vi "CE14_open handshake(subVI).vi"(8 "error in(no error)":errorcluster, 11 "VISA resource name":refnum<visa-resource-name>) -> (0 "error out":errorcluster, 1 "success":bool, 2 "response msg":string[](array[string]), 3 "VISA resource name 2":refnum<visa-resource-name>)   [LabVIEW 2018, in "CE14_eMIC.lvlib"]
uses:
  CE14_eMIC.lvlib
  type defs/CE14_state.ctl
  <vilib>/Instr/_visa.llb/VISA Configure Serial Port (Instr).vi
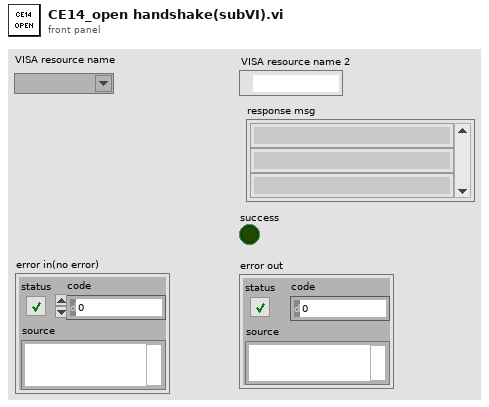
[diagram p1: front panel]
types:
  T1 = typedef "CE14_eMIC.lvlib/CE14_state.ctl" = enum16{"open COM (300)", "step1(300):2F 3F 21 0D 0A", "step2(300):06 30 34 31 0D 0A", "step3:Change4800", "step4(4800)", "stop"}
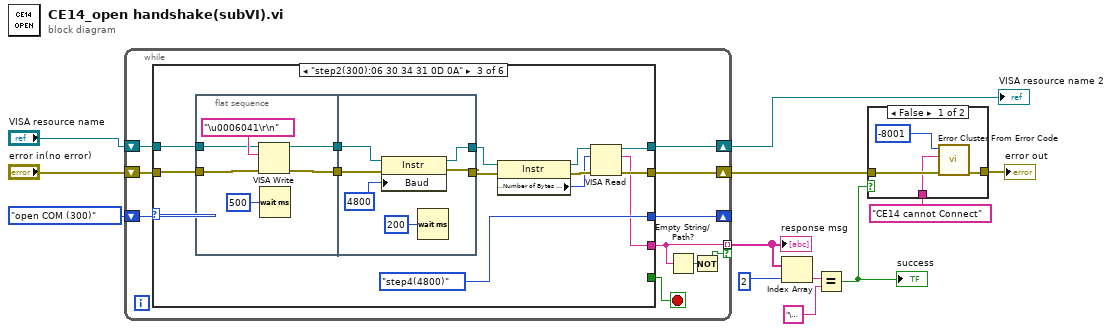
[diagram p0: block diagram]
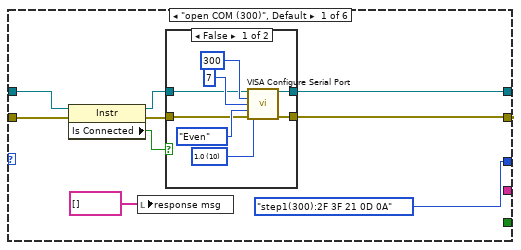
[diagram p3: hidden frame]
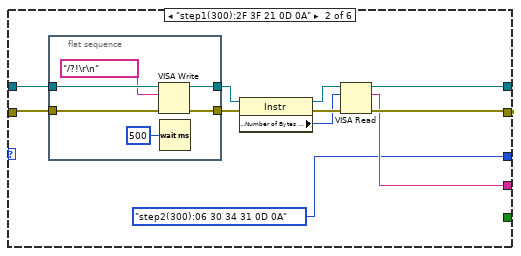
[diagram p5: hidden frame]
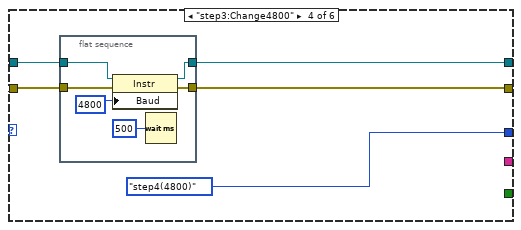
[diagram p6: hidden frame]
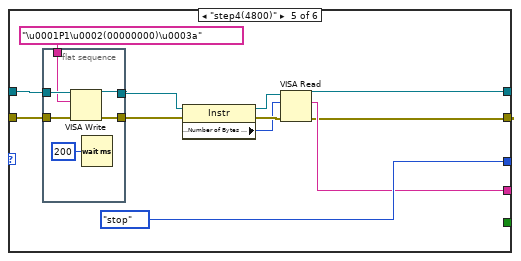
[diagram p7: hidden frame]
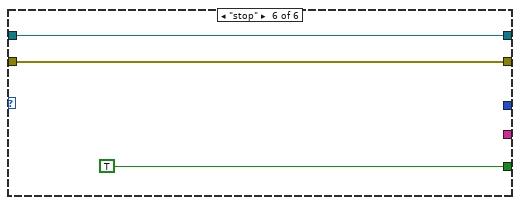
[diagram p8: hidden frame]
diagram:
  n1 = while {
    shift-right: [w21] -> w2
    shift-left: "VISA resource name" -> [w22]
    shift-right: [w20] -> w4
    shift-left: "error in(no error)" -> [w19]
    tunnel: [w17] -> w9 mode=indexing if=w13
    shift-right: [w16] -> _
    shift-left: CE14_state."open COM (300)" -> [w14]
    stop <- w15 stop-if-true
    n2 = case shown="\"step2(300):06 30 34 31 0D 0A\"" w14 {
      tunnel: w22 -> [w26 w52 w70 w88 w104 w114]
      tunnel: [w31 w45 w63 w85 w97 w114] -> w21
      tunnel: [w23 w47 w65 w86 w96 w113] -> w20
      tunnel: w19 -> [w30 w51 w71 w87 w103 w113]
      tunnel: [_ w43 w61 _ w105 _] -> w17
      tunnel: [CE14_state."step1(300):2F 3F 21 0D 0A" CE14_state."step2(300):06 30 34 31 0D 0A" CE14_state."step4(4800)" CE14_state."step4(4800)" CE14_state."stop" _] -> w16
      tunnel: [_ _ _ _ _ TRUE] -> w15
      frame "open COM (300)", Default {
        n3 = property class="Instr"(reference=w26, error in=w30) -> (reference out=w25:refnum<visa-resource-name>, error out=w27:errorcluster, "Is Connected"=w24:bool)
        n4 = local write "response msg"(string[] []) -> ()
        n5 = case shown="False" w24 {
          tunnel: [w35 w41] -> w31
          tunnel: [w34 w40] -> w23
          tunnel: w27 -> [w33 w40]
          tunnel: w25 -> [w32 w41]
          frame False {
            w36 = u16 10 items=["1.0"=10, "1.5"=15, "2.0"=20] ("stop bits (10: 1 bit)")
            n6 = call-poly "VISA Configure Serial Port"("VISA resource name"=w32, "baud rate (9600)"=u32 300, "data bits (8)"=u16 7, "parity (0:none)"=enum16{"None", "Odd", "Even", "Mark", "Space"}."Even", "error in (no error)"=w33, "stop bits (10: 1 bit)"=w36) -> ("VISA resource name out"=w35:refnum<visa-resource-name>, "error out"=w34:errorcluster)  [unwired: 8 in]
          }
          frame True {
          }
        }
      }
      frame "step1(300):2F 3F 21 0D 0A" {
        n7 = flat-sequence {
          tunnel: w52 -> [w58]
          tunnel: w51 -> [w57]
          tunnel: [w56] -> w50
          tunnel: [w55] -> w49
          frame #0 {
            n8 = VISA Write(VISA resource name=w58, write buffer="/?!\r\n", error in (no error)=w57) -> (VISA resource name out=w55:refnum<visa-resource-name>, error out=w56:errorcluster)  [unwired: 1 out]
            n9 = Wait (ms)(milliseconds to wait=u32 500) -> ()  [unwired: 1 out]
          }
        }
        n10 = property class="Instr"(reference=w49, error in=w50) -> (reference out=w46:refnum<visa-resource-name>, error out=w48:errorcluster, "Serial Settings:Number of Bytes at Serial Port"=w44:u32)
        n11 = VISA Read(VISA resource name=w46, byte count=w44, error in (no error)=w48) -> (VISA resource name out=w45:refnum<visa-resource-name>, read buffer=w43:string, error out=w47:errorcluster)  [unwired: 1 out]
      }
      frame "step2(300):06 30 34 31 0D 0A" {
        n12 = flat-sequence {
          tunnel: w70 -> [w73]
          tunnel: w71 -> [w72]
          tunnel: [w75] -> w60
          tunnel: [w74] -> w59
          tunnel: w60 -> [w80]
          tunnel: w59 -> [w79]
          tunnel: [w82] -> w68
          tunnel: [w81] -> w66
          frame #0 {
            n13 = VISA Write(VISA resource name=w73, write buffer="\u0006041\r\n", error in (no error)=w72) -> (VISA resource name out=w74:refnum<visa-resource-name>, error out=w75:errorcluster)  [unwired: 1 out]
            n14 = Wait (ms)(milliseconds to wait=u32 500) -> ()  [unwired: 1 out]
          }
          frame #1 {
            n15 = property class="Instr"(reference=w79, error in=w80, "Baud"=u32 4800 ("Serial Settings:Baud Rate")) -> (reference out=w81:refnum<visa-resource-name>, error out=w82:errorcluster)
            n16 = Wait (ms)(milliseconds to wait=u32 200) -> ()  [unwired: 1 out]
          }
        }
        n17 = property class="Instr"(reference=w66, error in=w68) -> (reference out=w64:refnum<visa-resource-name>, error out=w67:errorcluster, "Serial Settings:Number of Bytes at Serial Port"=w62:u32)
        n18 = VISA Read(VISA resource name=w64, byte count=w62, error in (no error)=w67) -> (VISA resource name out=w63:refnum<visa-resource-name>, read buffer=w61:string, error out=w65:errorcluster)  [unwired: 1 out]
      }
      frame "step3:Change4800" {
        n19 = flat-sequence {
          tunnel: w88 -> [w93]
          tunnel: w87 -> [w92]
          tunnel: [w91] -> w86
          tunnel: [w90] -> w85
          frame #0 {
            n20 = property class="Instr"(reference=w93, error in=w92, "Baud"=u32 4800 ("Serial Settings:Baud Rate")) -> (reference out=w90:refnum<visa-resource-name>, error out=w91:errorcluster)
            n21 = Wait (ms)(milliseconds to wait=u32 500) -> ()  [unwired: 1 out]
          }
        }
      }
      frame "step4(4800)" {
        n22 = flat-sequence {
          tunnel: w104 -> [w110]
          tunnel: w103 -> [w109]
          tunnel: "\u0001P1\u0002(00000000)\u0003a" ("write buffer") -> [w108]
          tunnel: [w112] -> w102
          tunnel: [w111] -> w99
          frame #0 {
            n23 = VISA Write(VISA resource name=w110, write buffer=w108, error in (no error)=w109) -> (VISA resource name out=w111:refnum<visa-resource-name>, error out=w112:errorcluster)  [unwired: 1 out]
            n24 = Wait (ms)(milliseconds to wait=u32 200) -> ()  [unwired: 1 out]
          }
        }
        n25 = property class="Instr"(reference=w99, error in=w102) -> (reference out=w100:refnum<visa-resource-name>, error out=w101:errorcluster, "Serial Settings:Number of Bytes at Serial Port"=w98:u32)
        n26 = VISA Read(VISA resource name=w100, byte count=w98, error in (no error)=w101) -> (VISA resource name out=w97:refnum<visa-resource-name>, read buffer=w105:string, error out=w96:errorcluster)  [unwired: 1 out]
      }
      frame "stop" {
      }
    }
    n27 = Empty String/Path?(string/path=w17) -> (empty?=w18:bool)
    n28 = Not(x=w18) -> (.not. x?=w13:bool)
  }
  "response msg" <- w9
  "VISA resource name 2" <- w2
  n29 = Index Array(array=w9, index=2) -> (element=w7:string)
  n30 = Equal?(x=w7, y="\u0006") -> (x = y?=w5:bool)
  "success" <- w5
  n31 = case shown="False" w5 {
    tunnel: w4 -> [w119 w120]
    tunnel: [w117 w120] -> w3
    tunnel: "CE14 cannot Connect" ("error message (\"\")") -> [w116 _]
    frame False {
      n32 = call <vilib>:"Error Cluster From Error Code.vi"("error in (no error)"=w119, "error message (\"\")"=w116, "error code (0)"=-8001) -> ("error out"=w117:errorcluster)  [unwired: 6 in]
    }
    frame True {
    }
  }
  "error out" <- w3
